vi "Set Task Base.vi"(8 "error in (no error)":errorcluster, 10 "HAL GOOP4.lvlib:Task Base.lvclass":refnum<class "Task Base.lvclass">, 11 "Task Actor in":refnum<class "Task Actor.lvclass">) -> (0 "error out":errorcluster, 3 "Task Actor out":refnum<class "Task Actor.lvclass">)   [LabVIEW 2023, in "Task Actor.lvlib" / "Task Actor.lvclass"]
uses:
  Task Actor.lvclass
  Task Actor.lvclass/Task Actor.ctl
  Task Base/Task Base.lvclass
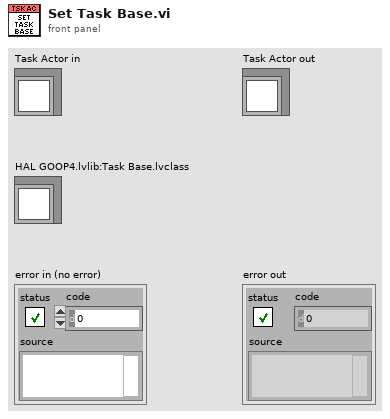
[diagram p1: front panel]
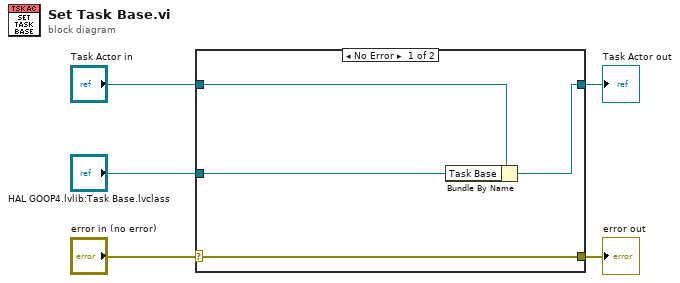
[diagram p0: block diagram]
diagram:
  n1 = case shown="No Error" "error in (no error)" {
    selector: "error in (no error)" -> [w9 w10]
    tunnel: [w9 w10] -> w4
    tunnel: [w7 w11] -> w2
    tunnel: "Task Actor in" -> [w8 w11]
    tunnel: "HAL GOOP4.lvlib:Task Base.lvclass" -> [w6 _]
    frame No Error {
      n2 = Bundle By Name(cluster=w8, "Task Base"=w6) -> (w7:refnum<class "Task Actor.lvclass">)
    }
    frame Error {
    }
  }
  "error out" <- w4
  "Task Actor out" <- w2
